vi "excelrowconcat_singlecol_LR_HR_2FILE.vi"() -> ()   [LabVIEW 2020]
uses:
  <vilib>/addons/_office/excel.llb/Excel Get Data ([dbl]).vi
  <vilib>/Utility/file.llb/Write To Spreadsheet File (DBL).vi
  <vilib>/Utility/NIReport.llb/NI_report.lvclass
  <vilib>/Utility/NIReport.llb/Excel/NI_Excel.lvclass
  <vilib>/addons/_office/NI_ReportGenerationToolkit.lvlib
panel:
  in  "Save row cutting file":bool
  out "Total LR Selected Row":i32=3
  in  "Tab Control":enum32{"HR", "LR", "RESULT"}(tab)
  out "HR selected row":ext[](array[numeric])=[5.0, 20.0, 35.0, 50.0] format="%#_6f"
  out "HR Sheet Values":ext[][](array[numeric])=[[1.0, 16.0, 31.0, 46.0], [2.0, 17.0, 32.0, 47.0], [3.0, 18.0, 33.0, 48.0], [4.0, 19.0, 34.0, 49.0], [5.0, 20.0, 35.0, 50.0], [6.0, 21.0, 36.0, 51.0], [7.0, 22.0, 37.0, 52.0], [8.0, 23.0, 38.0, 53.0], [9.0, 24.0, 39.0, 54.0], [10.0, 25.0, 40.0, 55.0], [11.0, 26.0, 41.0, 56.0], [12.0, 27.0, 42.0, 57.0], [13.0, 28.0, 43.0, 58.0], [14.0, 29.0, 44.0, 59.0], [15.0, 30.0, 45.0, 60.0]] format="%_6f"
  out "HR Added row":ext[][](array[numeric])=[[1.0, 16.0, 31.0, 46.0], [3.0, 18.0, 33.0, 48.0], [5.0, 20.0, 35.0, 50.0]] format="%#_6f"
  out "HR Selected Column":ext[](array[numeric])=[46.0, 48.0, 50.0] format="%#_6f"
  out "HR Stack Col":ext[](array[numeric])=[1.0, 3.0, 5.0, 16.0, 18.0, 20.0, 31.0, 33.0, 35.0, 46.0, 48.0, 50.0] format="%#_6f"
  out "Rows":i32=15
  out "Columns":i32=4
  out "LR selected row":ext[](array[numeric])=[6.0, 21.0, 36.0, 51.0] format="%#_6f"
  out "LR Sheet Values":ext[][](array[numeric])=[[1.0, 16.0, 31.0, 46.0], [2.0, 17.0, 32.0, 47.0], [3.0, 18.0, 33.0, 48.0], [4.0, 19.0, 34.0, 49.0], [5.0, 20.0, 35.0, 50.0], [6.0, 21.0, 36.0, 51.0], [7.0, 22.0, 37.0, 52.0], [8.0, 23.0, 38.0, 53.0], [9.0, 24.0, 39.0, 54.0], [10.0, 25.0, 40.0, 55.0], [11.0, 26.0, 41.0, 56.0], [12.0, 27.0, 42.0, 57.0], [13.0, 28.0, 43.0, 58.0], [14.0, 29.0, 44.0, 59.0], [15.0, 30.0, 45.0, 60.0]] format="%_6f"
  out "LR Added row":ext[][](array[numeric])=[[2.0, 17.0, 32.0, 47.0], [4.0, 19.0, 34.0, 49.0], [6.0, 21.0, 36.0, 51.0]] format="%#_6f"
  out "LR Selected Column":ext[](array[numeric])=[47.0, 49.0, 51.0] format="%#_6f"
  out "LR Stack Col":ext[](array[numeric])=[2.0, 4.0, 6.0, 17.0, 19.0, 21.0, 32.0, 34.0, 36.0, 47.0, 49.0, 51.0] format="%#_6f"
  out "HR_LR":ext[][](array[numeric])=[[1.0, 2.0], [3.0, 4.0], [5.0, 6.0], [16.0, 17.0], [18.0, 19.0], [20.0, 21.0], [31.0, 32.0], [33.0, 34.0], [35.0, 36.0], [46.0, 47.0], [48.0, 49.0], [50.0, 51.0]]
  in  "LR state  Row Number (2,4)":string="2,4,6"
  in  "Excel._Worksheet":refnum<k7>
  in  "Excel._Application":refnum<k7>
  in  "precission":string="6"
  in  "Destination path for cutting rows":path=path "C:/Users/lab user/Desktop/cm/single column"
  in  "row cut file name (no extension)":string="SCDUAL"
  in  "HR state  Row Number (1,3)":string="1,3,5"
  out "Total HR Selected Row":i32=3
  in  "Select Excel file":path=path "C:/Users/lab user/Desktop/cm/single column/sc.xls"
  # "HR column stack output will be save in same directory\nrow cut file name_HR_LR_single_col.xls"
  # "HR Row cut output will be save in same directory\nrow cut file name_HR.xls"
  # "LR Row cut  output will be save in same directory\nrow cut file name_LR.xls"
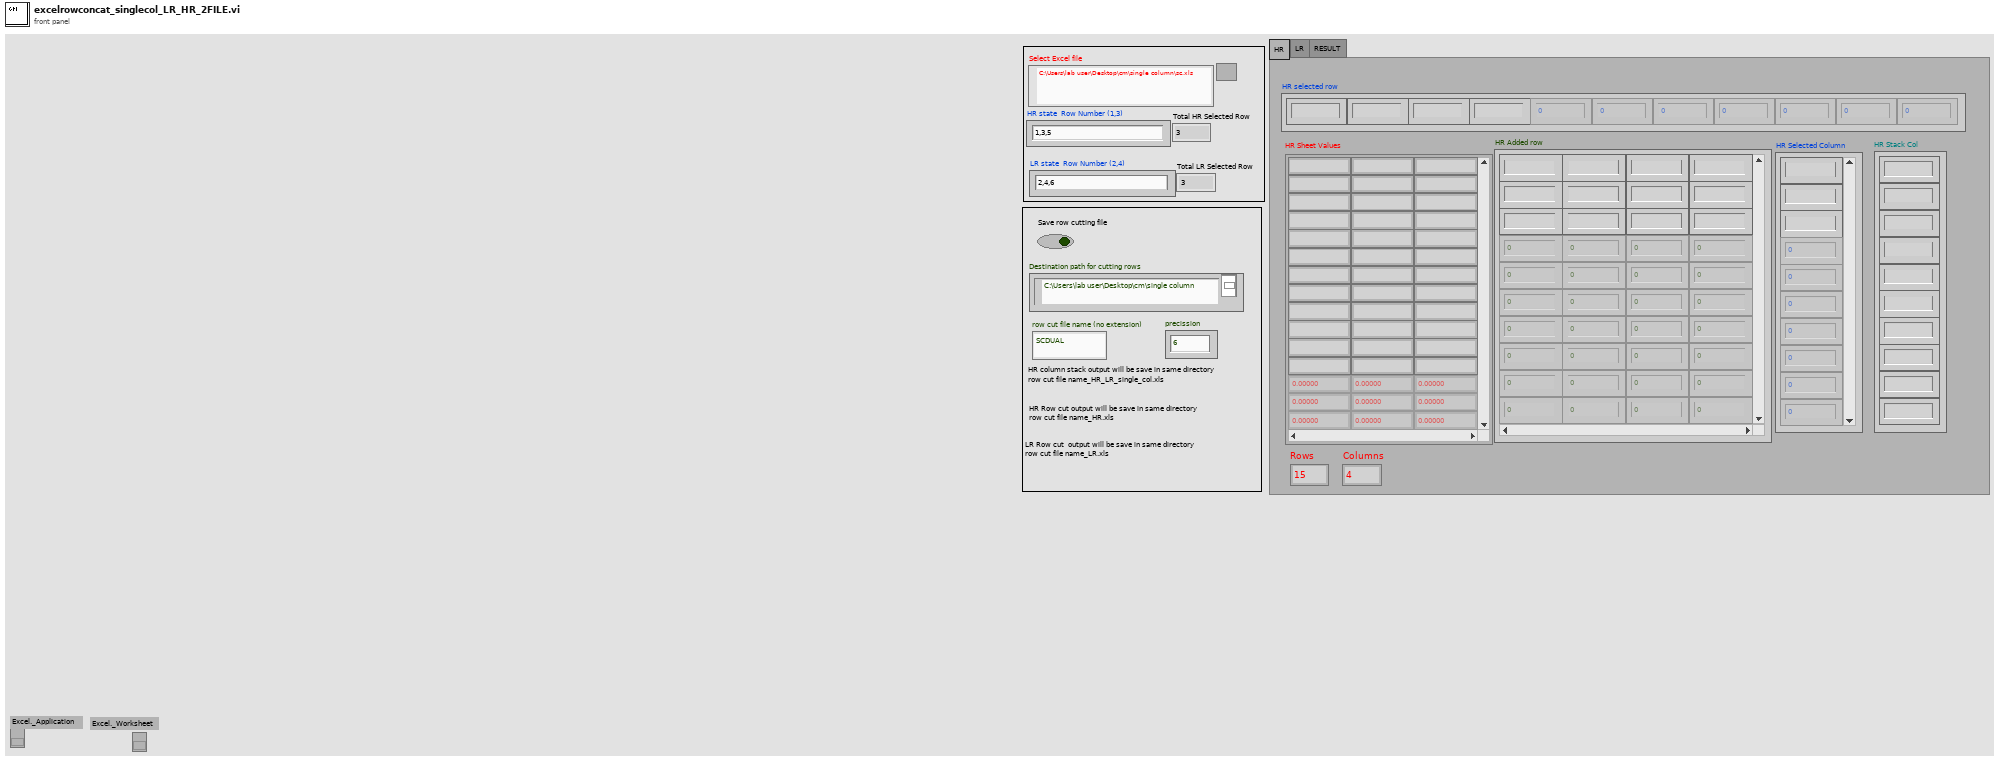
[diagram p1: front panel]
types:
  T1 = enum16{"Standard Report", "HTML", "Word", "Excel"}
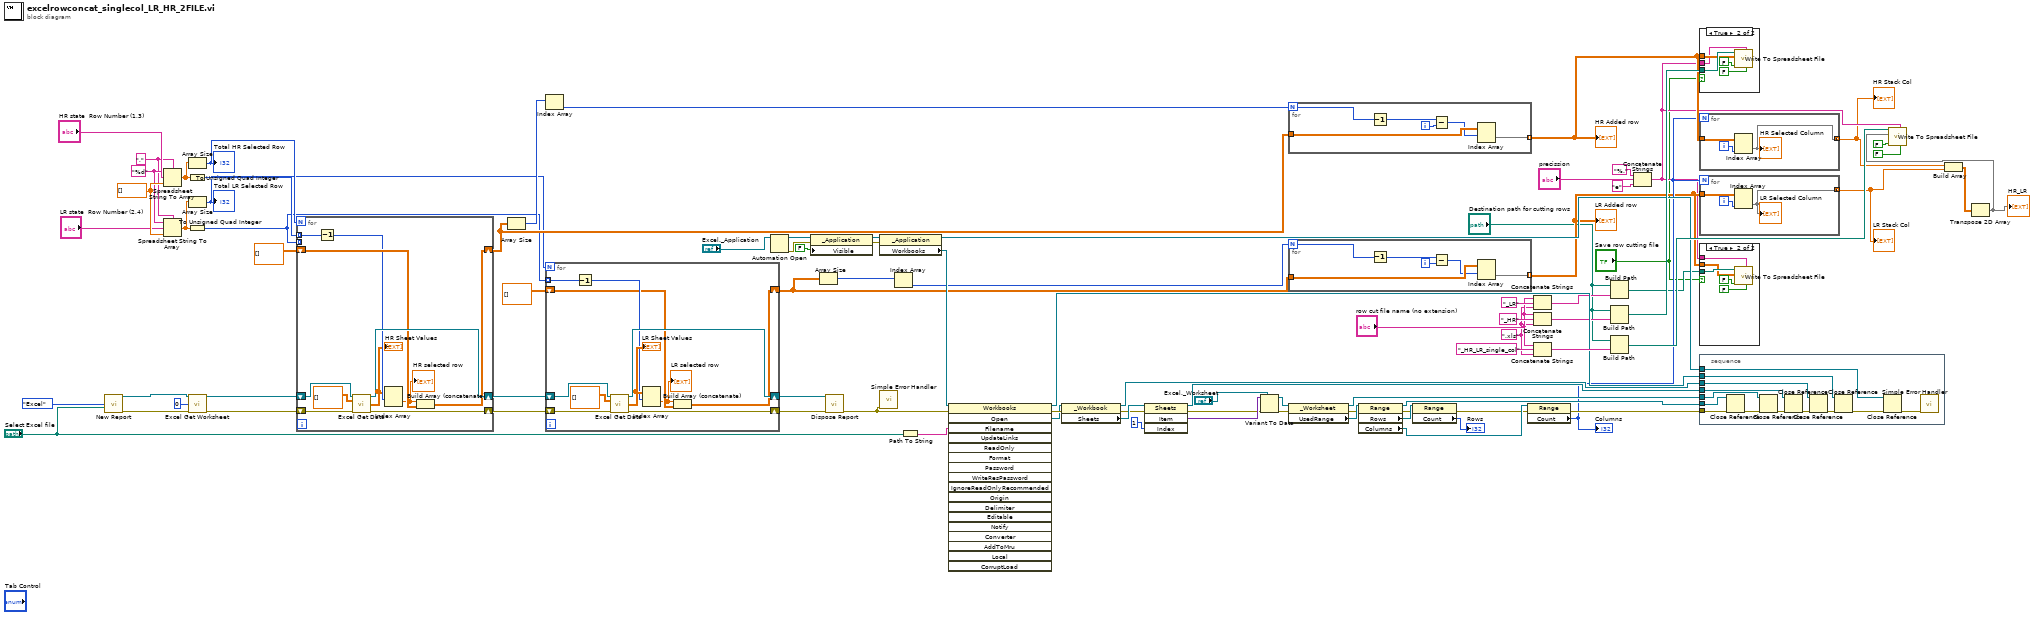
[diagram p0: block diagram]
diagram:
  w17 = ".xls" ("string")
  w32 = dbl[] []
  w29 = "," ("delimiter (Tab)")
  w30 = "%d" ("format string")
  n1 = call <vilib>:"New Report.vi"("report type"=T1."Excel", "template (empty)"="Select Excel file") -> ("report out"=w82:refnum<class "NI_report.lvclass">, "error out"=w83:errorcluster)  [unwired: 12 in]
  n2 = Spreadsheet String To Array(delimiter (Tab)=w29, format string=w30, spreadsheet string="HR state  Row Number (1,3)", array type (2D Dbl)=w32) -> (array=w86:dbl[])
  n3 = Spreadsheet String To Array(delimiter (Tab)=w29, format string=w30, spreadsheet string="LR state  Row Number (2,4)", array type (2D Dbl)=w32) -> (array=w16:dbl[])
  n4 = To Unsigned Quad Integer(1:w86) -> (0:w85:u64[])
  n5 = To Unsigned Quad Integer(1:w16) -> (0:w14:u64[])
  n6 = Array Size(array=w86) -> (size(s)=w67:i32)
  "Total HR Selected Row" <- w67
  n7 = Array Size(array=w16) -> (size(s)=w11:i32)
  "Total LR Selected Row" <- w11
  n8 = call <vilib>:"Excel Get Worksheet.vi"("report in"=w82, "worksheet index (0)"=0, "error in (no error)"=w83) -> ("report out"=w15:refnum<class "NI_report.lvclass">, "error out"=w81:errorcluster)  [unwired: 11 in]
  n9 = for {
    N: w67 -> [_]
    shift-right: [w99] -> w9
    shift-left: w15 -> [w94]
    shift-right: [w98] -> w8
    shift-left: w81 -> [w95]
    shift-right: [w96] -> w80
    shift-left: ext[][] [] -> [w97]
    tunnel: w85 -> [w93] mode=indexing
    tunnel: w14 -> [_] mode=indexing
    n10 = Decrement(x=w93) -> (x-1=w92:u64)
    n11 = call-poly <vilib>:"Excel Get Data.vi"("report in"=w94, "data type"=ext[][] [], "error in (no error)"=w95) -> ("report out"=w99:refnum<class "NI_report.lvclass">, "data"=w90:dbl[][], "error out"=w98:errorcluster)  [unwired: 10 in]
    "HR Sheet Values" <- w90
    n12 = Index Array(array=w90, index (row)=w92) -> (element=w91:dbl[])  [unwired: 1 in]
    "HR selected row" <- w91
    n13 = Build Array (concatenate)(w91, w97) -> (w96:ext[][])
  }
  n14 = Array Size(array=w80) -> (size(s)=w78:i32[])
  n15 = Index Array(array=w78) -> (element=w79:i32)  [unwired: 1 in]
  n16 = for {
    N: w11 -> [_]
    shift-right: [w110] -> w7
    shift-left: w9 -> [w107]
    shift-right: [w109] -> w6
    shift-left: w8 -> [w108]
    tunnel: w14 -> [w105] mode=indexing
    shift-right: [w103] -> w13
    shift-left: ext[][] [] -> [w102]
    n17 = Decrement(x=w105) -> (x-1=w104:u64)
    n18 = call-poly <vilib>:"Excel Get Data.vi"("report in"=w107, "data type"=ext[][] [], "error in (no error)"=w108) -> ("report out"=w110:refnum<class "NI_report.lvclass">, "data"=w106:dbl[][], "error out"=w109:errorcluster)  [unwired: 10 in]
    "LR Sheet Values" <- w106
    n19 = Index Array(array=w106, index (row)=w104) -> (element=w101:dbl[])  [unwired: 1 in]
    "LR selected row" <- w101
    n20 = Build Array (concatenate)(w101, w102) -> (w103:ext[][])
  }
  n21 = Automation Open(Automation Refnum="Excel._Application") -> (Automation Refnum=w59:refnum<k7>, error out=w62:errorcluster)  [unwired: 3 in]
  n22 = property class="_Application"(reference=w59, error in=w62, "Visible"=FALSE ("Make Excel Visible")) -> (reference out=w58:refnum<k7>, error out=w61:errorcluster)
  n23 = Array Size(array=w13) -> (size(s)=w27:i32[])
  n24 = call-dynamic "Dispose Report.vi"("report in"=w7, "error in (no error)"=w6) -> ("error out"=w35:errorcluster)  [unwired: 13 in]
  n25 = property class="_Application"(reference=w58, error in=w61) -> (reference out=w44:refnum<k7>, "Workbooks"=w47:refnum<k7>)  [unwired: 1 out]
  n26 = call <vilib>:"Simple Error Handler.vi"("error in (no error)"=w35) -> ()  [unwired: 4 in, 5 out]
  n27 = Index Array(array=w27) -> (element=w26:i32)  [unwired: 1 in]
  n28 = Path To String(path="Select Excel file") -> (string=w36:string)
  n29 = invoke class="Workbooks" method="Open"(reference=w47, error in=w35, "Filename"=w36) -> (reference out=w43:refnum<k7>, error out=w65:errorcluster, "Open"=w53:refnum<k7>)  [unwired: 15 in, 15 out]
  n30 = property class="_Workbook"(reference=w53, error in=w65) -> (reference out=w42:refnum<k7>, error out=w52:errorcluster, "Sheets"=w54:refnum<k7>)
  n31 = invoke class="Sheets" method="Item"(reference=w54, error in=w52, "Index"=1) -> (reference out=w41:refnum<k7>, error out=w51:errorcluster, "Item"=w64:variant)  [unwired: 1 in, 1 out]
  n32 = Variant To Data(error in=w51, type="Excel._Worksheet", Variant=w64) -> (data=w55:refnum<k7>, error out=w50:errorcluster)
  n33 = for {
    N: w79 -> [w117]
    tunnel: w80 -> [w114]
    tunnel: [w112] -> w73 mode=indexing
    i -> [w115]
    n34 = Decrement(x=w117) -> (x-1=w116:i32)
    n35 = Subtract(x=w116, y=w115) -> (x-y=w113:i32)
    n36 = Index Array(array=w114, index (row)=w113) -> (element=w112:ext[])  [unwired: 1 in]
  }
  "HR Added row" <- w73
  n37 = for {
    N: w26 -> [w123]
    tunnel: w13 -> [w120]
    tunnel: [w118] -> w20 mode=indexing
    i -> [w121]
    n38 = Decrement(x=w123) -> (x-1=w122:i32)
    n39 = Subtract(x=w122, y=w121) -> (x-y=w119:i32)
    n40 = Index Array(array=w120, index (row)=w119) -> (element=w118:ext[])  [unwired: 1 in]
  }
  "LR Added row" <- w20
  n41 = property class="_Worksheet"(reference=w55, error in=w50) -> (reference out=w40:refnum<k7>, error out=w49:errorcluster, "UsedRange"=w56:refnum<k7>)
  n42 = property class="Range"(reference=w56, error in=w49) -> (reference out=w39:refnum<k7>, error out=w48:errorcluster, "Rows"=w57:refnum<k7>, "Columns"=w45:refnum<k7>)
  n43 = property class="Range"(reference=w57, error in=w48) -> (error out=w38:errorcluster, "Count"=→"Rows":i32)  [unwired: 1 out]
  n44 = property class="Range"(reference=w45, error in=w38) -> (error out=w37:errorcluster, "Count"=w25:i32)  [unwired: 1 out]
  "Columns" <- w25
  n45 = Concatenate Strings("row cut file name (no extension)", "_LR" ("string"), w17) -> (w22:string)
  n46 = Concatenate Strings("row cut file name (no extension)", "_HR" ("string"), w17) -> (w33:string)
  n47 = Concatenate Strings("row cut file name (no extension)", "_HR_LR_single_col" ("string"), w17) -> (w68:string)
  n48 = Build Path(base path="Destination path for cutting rows", name or relative path=w22) -> (appended path=w21:path)
  n49 = Build Path(base path="Destination path for cutting rows", name or relative path=w33) -> (appended path=w77:path)
  n50 = Build Path(base path="Destination path for cutting rows", name or relative path=w68) -> (appended path=w70:path)
  n51 = Concatenate Strings("%.", "precission", "e") -> (w10:string)
  n52 = case shown="True" "Save row cutting file" {
    tunnel: w77 -> [_ w126]
    tunnel: w73 -> [_ w125]
    tunnel: w10 -> [_ w124]
    frame False {
    }
    frame True {
      n53 = call-poly <vilib>:"Write To Spreadsheet File.vi"("transpose? (no:F)"=FALSE, "format (%.3f)"=w124, "append to file? (new file:F)"=FALSE, "2D data"=w125, "file path (dialog if empty)"=w126) -> ()  [unwired: 3 in, 1 out]
    }
  }
  n54 = for {
    N: w25 -> [_]
    tunnel: w73 -> [w130]
    tunnel: [w129] -> w4 mode=concatenating
    i -> [w131]
    n55 = Index Array(array=w130, index (col)=w131) -> (element=w129:ext[])  [unwired: 1 in]
    "HR Selected Column" <- w129
  }
  "HR Stack Col" <- w4
  n56 = for {
    N: w25 -> [_]
    tunnel: w20 -> [w133]
    tunnel: [w132] -> w3 mode=concatenating
    i -> [w134]
    n57 = Index Array(array=w133, index (col)=w134) -> (element=w132:ext[])  [unwired: 1 in]
    "LR Selected Column" <- w132
  }
  "LR Stack Col" <- w3
  n58 = case shown="True" "Save row cutting file" {
    tunnel: w21 -> [_ w137]
    tunnel: w20 -> [_ w136]
    tunnel: w10 -> [_ w135]
    frame False {
    }
    frame True {
      n59 = call-poly <vilib>:"Write To Spreadsheet File.vi"("transpose? (no:F)"=FALSE, "format (%.3f)"=w135, "append to file? (new file:F)"=FALSE, "2D data"=w136, "file path (dialog if empty)"=w137) -> ()  [unwired: 3 in, 1 out]
    }
  }
  n60 = stacked-sequence {
    tunnel: w44 -> [w152]
    tunnel: w43 -> [w151]
    tunnel: w42 -> [w150]
    tunnel: w41 -> [w149]
    tunnel: w40 -> [w148]
    tunnel: w39 -> [w147]
    tunnel: w37 -> [w146]
    frame #0 {
      n61 = Close Reference(reference=w147, error in (no error)=w146) -> (error out=w145:errorcluster)
      n62 = Close Reference(reference=w148, error in (no error)=w145) -> (error out=w144:errorcluster)
      n63 = Close Reference(reference=w149, error in (no error)=w144) -> (error out=w143:errorcluster)
      n64 = Close Reference(reference=w150, error in (no error)=w143) -> (error out=w142:errorcluster)
      n65 = Close Reference(reference=w151, error in (no error)=w142) -> (error out=w141:errorcluster)
      n66 = Close Reference(reference=w152, error in (no error)=w141) -> (error out=w140:errorcluster)
      n67 = call <vilib>:"Simple Error Handler.vi"("error in (no error)"=w140) -> ()  [unwired: 4 in, 5 out]
    }
  }
  n68 = Build Array(w4, w3) -> (w2:ext[][])
  n69 = Transpose 2D Array(2D array=w2) -> (transposed array=w1:ext[][])
  "HR_LR" <- w1
  n70 = call-poly <vilib>:"Write To Spreadsheet File.vi"("transpose? (no:F)"=FALSE, "format (%.3f)"=w10, "append to file? (new file:F)"=FALSE, "2D data"=w1, "file path (dialog if empty)"=w70) -> ()  [unwired: 3 in, 1 out]
